vi "test_BuildAdvancedAssets_TargetsDifferentCompilersAdvanced.vi"() -> (0 "error out":errorcluster, 3 "Pass?":bool)   [LabVIEW 2019, in "Tests.SolutionBuilder.lvlib"]
uses:
  Tests.SolutionBuilder.lvlib
  SolutionBuilder/SolutionBuilder.lvclass
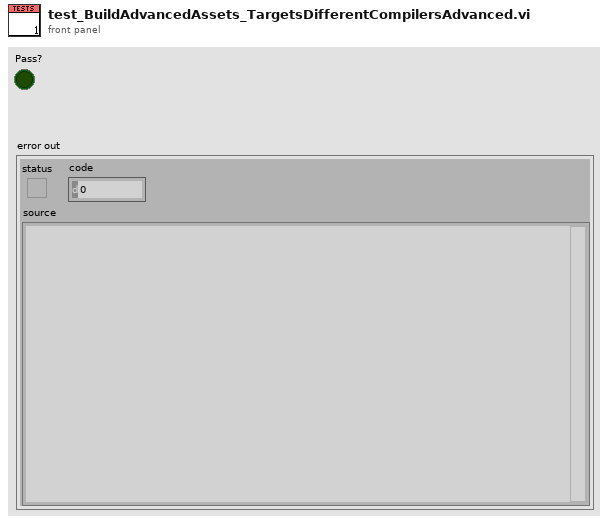
[diagram p1: front panel]
types:
  T1 = typedef "SolutionBuilder.lvlib/BuildManager.lvclass/GeneratedFile.ctl" = map{cluster{"Project path":string, "Build spec name":string}, set{string}}
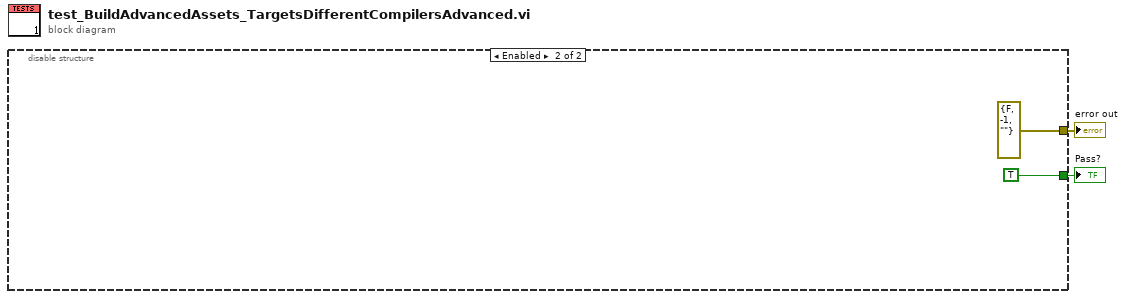
[diagram p0: block diagram]
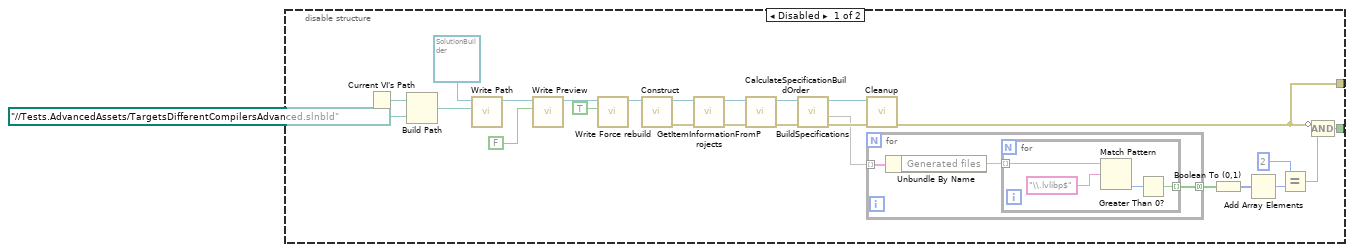
[diagram p2: hidden frame]
diagram:
  n1 = disable-structure shown="Enabled" {
    disable-tunnel: [w27 TRUE ("Pass?")] -> w2
    disable-tunnel: [w12 errorcluster {"status"=FALSE, "code"=-1, "source"=""} ("error out")] -> w1
    frame Disabled {
      n2 = Current VI's Path() -> (path=w25:path)
      n3 = Build Path(base path=w25, name or relative path=path "../../Tests.AdvancedAssets/TargetsDifferentCompilersAdvanced.slnbld" ("Path")) -> (appended path=w23:path)
      n4 = call "Write Path.vi"("Path"=w23, "SolutionBuilder in"=refnum<class "SolutionBuilder.lvclass"> refnum) -> ("SolutionBuilder out"=w14:refnum<class "SolutionBuilder.lvclass">)  [unwired: 9 in]
      n5 = call "Write Preview.vi"("Preview?"=FALSE, "SolutionBuilder in"=w14) -> ("SolutionBuilder out"=w5:refnum<class "SolutionBuilder.lvclass">)  [unwired: 9 in]
      n6 = call "Write Force rebuild.vi"("Force rebuild"=TRUE, "SolutionBuilder in"=w5) -> ("SolutionBuilder out"=w4:refnum<class "SolutionBuilder.lvclass">)  [unwired: 9 in]
      n7 = call "Construct.vi"("SolutionBuilder in"=w4) -> ("error out"=w19:errorcluster, "SolutionBuilder out"=w22:refnum<class "SolutionBuilder.lvclass">)  [unwired: 9 in]
      n8 = call "GetItemInformationFromProjects.vi"("error in (no error)"=w19, "SolutionBuilder in"=w22) -> ("error out"=w18:errorcluster, "SolutionBuilder out"=w21:refnum<class "SolutionBuilder.lvclass">)  [unwired: 8 in]
      n9 = call "CalculateSpecificationBuildOrder.vi"("error in (no error)"=w18, "SolutionBuilder in"=w21) -> ("error out"=w17:errorcluster, "SolutionBuilder out"=w20:refnum<class "SolutionBuilder.lvclass">)  [unwired: 8 in]
      n10 = call "BuildSpecifications.vi"("error in (no error)"=w17, "SolutionBuilder in"=w20) -> ("error out"=w16:errorcluster, "Generated file"=w7:T1, "SolutionBuilder out"=w15:refnum<class "SolutionBuilder.lvclass">)  [unwired: 7 in]
      n11 = call "Cleanup.vi"("error in (no error)"=w16, "SolutionBuilder in"=w15) -> ("error out"=w12:errorcluster)  [unwired: 8 in, 1 out]
      n12 = for {
        tunnel: w7 -> [w30] mode=indexing
        tunnel: [w28] -> w6 mode=concatenating
        n13 = Unbundle By Name(w30) -> ("Generated files"=w29:set{string})
        n14 = for {
          tunnel: w29 -> [w31] mode=indexing
          tunnel: [w32] -> w28 mode=indexing
          n15 = Match Pattern(string=w31, regular expression="\\.lvlibp$") -> (offset past match=w33:i32)  [unwired: 1 in, 3 out]
          n16 = Greater Than 0?(x=w33) -> (x > 0?=w32:bool)
        }
      }
      n17 = Boolean To (0,1)(Boolean=w6) -> (0, 1=w9:i16[])
      n18 = Add Array Elements(numeric array=w9) -> (sum=w8:i16)
      n19 = Equal?(x=i16 2, y=w8) -> (x = y?=w10:bool)
      n20 = Compound Arithmetic op=AND(invert w12, w10) -> (w27:bool)
    }
    frame Enabled {
    }
  }
  "Pass?" <- w2
  "error out" <- w1
